vi "Getcontrolreferences.vi"(11 "reference":refnum<vi>) -> (2 "filepath control ref":refnum<vi>, 3 "stop control ref":refnum<vi>)   [LabVIEW 2018]
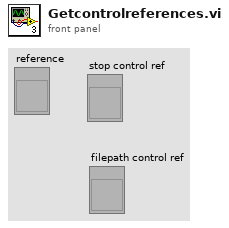
[diagram p1: front panel]
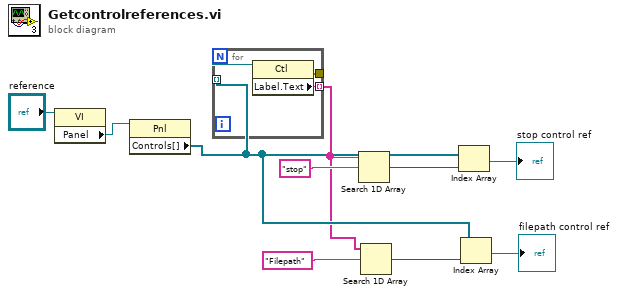
[diagram p0: block diagram]
diagram:
  n1 = property class="VI"(reference="reference") -> ("Panel"=w8:refnum<vi>)  [unwired: 1 in, 2 out]
  n2 = property class="Pnl"(reference=w8) -> ("Controls[]"=w2:refnum<vi>[])  [unwired: 1 in, 2 out]
  n3 = for {
    tunnel: w2 -> [w13] mode=indexing
    tunnel: [w12] -> w1 mode=indexing
    tunnel: [w11] -> _
    n4 = property class="Ctl"(reference=w13) -> (error out=w11:errorcluster, "Label.Text"=w12:string)  [unwired: 1 in, 1 out]
  }
  n5 = Search 1D Array(1D array=w1, element="stop") -> (index of element=w7:i32)  [unwired: 1 in]
  n6 = Search 1D Array(1D array=w1, element="Filepath") -> (index of element=w5:i32)  [unwired: 1 in]
  n7 = Index Array(array=w2, index=w7) -> (element=→"stop control ref":refnum<vi>)
  n8 = Index Array(array=w2, index=w5) -> (element=→"filepath control ref":refnum<vi>)
